vi "Stop Core.vi"(10 "final error code":i32, 11 "CS++RTMainActor in":refnum<class "CS++RTMainActor.lvclass">) -> (3 "CS++RTMainActor out":refnum<class "CS++RTMainActor.lvclass">)   [LabVIEW 2014, in "CS++RTMain.lvlib" / "CS++RTMainActor.lvclass"]
doc: "(<B>Filename</B>: Actor Framework.lvlib:Actor.lvclass:Stop Core.vi)\n\nDefines what the actor does before it stops. Use the <B>final error code</B> input to determine whether the actor shut down in response to an error.\n\nBy default, this method does nothing. A descendant class may override it to define behavior, such as shutting down any processes the actor initiated in its override of the Actor Core method."
uses:
  CS++RTMainActor.lvclass
  <vilib>/ActorFramework/Actor/Actor.lvclass
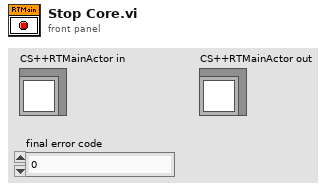
[diagram p1: front panel]
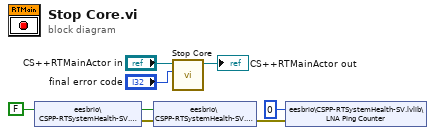
[diagram p0: block diagram]
diagram:
  w3 = FALSE
  n1 = shared-variable "eesbrio\\CSPP-RTSystemHealth-SV.lvlib\\LNA Reader"(w3) -> (error out=w4:errorcluster)  [unwired: 1 in]
  n2 = shared-variable "eesbrio\\CSPP-RTSystemHealth-SV.lvlib\\LNA Writer"(w3, error in=w4) -> (error out=w2:errorcluster)
  n3 = call-parent "Stop Core.vi"("final error code"="final error code", "Actor in"="CS++RTMainActor in") -> ("Actor out"=→"CS++RTMainActor out":refnum<class "CS++RTMainActor.lvclass">)  [unwired: 9 in]
  n4 = shared-variable "eesbrio\\CSPP-RTSystemHealth-SV.lvlib\\LNA Ping Counter"(u64 0 ("LNA Ping Counter"), error in=w2) -> ()  [unwired: 1 out]
